vi "MNIST_Classifier(Deploy).vi"() -> ()   [LabVIEW 2024]
doc: "Overview: This example demonstrates the usage of Deep Learning Toolkit for loading the model pre-trained for handwritten digit recognition and running for inference.\nRequirements: Deep Learning Toolkit for LabVIEW."
uses:
  <vilib>/Ngene/Deep Learning Toolkit/Toolkit/NN_Network/Controls/NN_Device.ctl
  <vilib>/Ngene/Deep Learning Toolkit/Toolkit/NN_Network/Controls/NN_Save_Before_Destroy_Options.ctl
  <extravilib>/ChannelInstances/Tag-bool/Write With Abort.vi
  <extravilib>/ChannelInstances/Tag-bool/Read With Abort.vi
  <extravilib>/ChannelInstances/Tag-bool/Instantiate.vi
  <extravilib>/ChannelInstances/Tag-bool/EndpointRead.vi
  <vilib>/Ngene/Deep Learning Toolkit/Toolkit/NN_Network/API/NN_Set_Input/3D/NN_Set_Input(3D_SGL_idx).vi
  <extravilib>/ChannelInstances/Tag-bool/Endpoint.vi
  <vilib>/Ngene/Deep Learning Toolkit/Toolkit/Deep_Learning_Toolkit_by_Ngene.lvlib
  <extravilib>/ChannelInstances/Tag-bool.lvlib
panel:
  in  "Pen Width":dbl
  out "Labels":string[](array[string])=["0", "1", "2", "3", "4", "5", "6", "7", "8", "9"]
  in  "Network Configuration File Path":path
  in  "Weight File Path":path
  out "Pen Attributes":T1={"Width"=24, "Style"=enum."Solid"}
  out "Draw Digit (280x280 px)":picture
  in  "Pen Color":u32(colorbox)=197379
  in  "Clear":bool
  out "Test Speed (img/s)":dbl=2316.9601485204007 format="%#_3p"
  out "test time(s/img)":dbl=0.00043159999995623366 format="%#_3p"
  out "Predictions":sgl[](array[slide])=[0.00022317072, 0.0016224136, 0.00590554, 0.9895844, 0.0010204009, 0.00023260966, 0.00083900435, 0.00020435848, 0.00020539068, 0.00016265694] scale=0.0..1.0
  in  "Pen Width":dbl=24.0
  in  "Stop Test":bool
  out "image (28x28px)":sgl[][](graph)=[[-1.0, -1.0, -1.0, -1.0, -1.0, -1.0, -1.0, -1.0, -1.0, -1.0, -1.0, -1.0, -1.0, -1.0, -1.0, -1.0, -1.0, -1.0, -1.0, -1.0, -1.0, -1.0, -1.0, -1.0, -1.0, -1.0, -1.0, -1.0], [-1.0, -1.0, -1.0, -1.0, -1.0, -1.0, -1.0, -1.0, -1.0, -1.0, -1.0, -1.0, -1.0, -1.0, -1.0, -1.0, -1.0, -1.0, -1.0, -1.0, -1.0, -1.0, -1.0, -1.0, -1.0, -1.0, -1.0, -1.0], [-1.0, -1.0, -1.0, -1.0, -1.0, -1.0, -1.0, -1.0, -0.81929135, -0.2570866, -0.33740157, -0.6988189, -1.0, -1.0, -1.0, -1.0, -1.0, -1.0, -1.0, -1.0, -1.0, -1.0, -1.0, -1.0, -1.0, -1.0, -1.0, -1.0], [-1.0, -1.0, -1.0, -1.0, -1.0, -1.0, -1.0, -0.19685039, 0.9476378, 1.007874, 1.007874, 0.9877953, 0.024015749, -1.0, -1.0, -1.0, -1.0, -1.0, -1.0, -1.0, -1.0, -1.0, -1.0, -1.0, -1.0, -1.0, -1.0, -1.0], [-1.0, -1.0, -1.0, -1.0, -1.0, -1.0, -1.0, 0.32519686, 1.007874, 1.007874, 1.007874, 1.007874, 1.007874, -0.21692914, -1.0, -1.0, -1.0, -1.0, -1.0, -1.0, -1.0, -1.0, -1.0, -1.0, -1.0, -1.0, -1.0, -1.0], [-1.0, -1.0, -1.0, -1.0, -1.0, -1.0, -1.0, -0.81929135, -0.19685039, -0.67874014, -0.71889764, 0.72677165, 1.007874, 0.78700787, -0.9799213, -1.0, -1.0, -1.0, -1.0, -1.0, -1.0, -1.0, -1.0, -1.0, -1.0, -1.0, -1.0, -1.0], [-1.0, -1.0, -1.0, -1.0, -1.0, -1.0, -1.0, -1.0, -1.0, -1.0, -1.0, -0.2972441, 1.007874, 1.007874, -0.6586614, -1.0, -1.0, -1.0, -1.0, -1.0, -1.0, -1.0, -1.0, -1.0, -1.0, -1.0, -1.0, -1.0], [-1.0, -1.0, -1.0, -1.0, -1.0, -1.0, -1.0, -1.0, -1.0, -1.0, -1.0, -0.5984252, 1.007874, 1.007874, -0.45787403, -1.0, -1.0, -1.0, -1.0, -1.0, -1.0, -1.0, -1.0, -1.0, -1.0, -1.0, -1.0, -1.0], [-1.0, -1.0, -1.0, -1.0, -1.0, -1.0, -1.0, -1.0, -1.0, -1.0, -1.0, -0.5984252, 1.007874, 1.007874, -0.5582677, -1.0, -1.0, -1.0, -1.0, -1.0, -1.0, -1.0, -1.0, -1.0, -1.0, -1.0, -1.0, -1.0], [-1.0, -1.0, -1.0, -1.0, -1.0, -1.0, -1.0, -1.0, -1.0, -1.0, -1.0, -0.19685039, 1.007874, 1.007874, -0.6185039, -1.0, -1.0, -1.0, -1.0, -1.0, -1.0, -1.0, -1.0, -1.0, -1.0, -1.0, -1.0, -1.0], [-1.0, -1.0, -1.0, -1.0, -1.0, -1.0, -1.0, -1.0, -1.0, -1.0, -0.19685039, 0.9476378, 1.007874, 0.62637794, -0.9799213, -1.0, -1.0, -1.0, -1.0, -1.0, -1.0, -1.0, -1.0, -1.0, -1.0, -1.0, -1.0, -1.0], [-1.0, -1.0, -1.0, -1.0, -1.0, -1.0, -1.0, -0.8996063, 0.3051181, 0.72677165, 1.007874, 1.007874, 1.007874, -0.23700787, -1.0, -1.0, -1.0, -1.0, -1.0, -1.0, -1.0, -1.0, -1.0, -1.0, -1.0, -1.0, -1.0, -1.0], [-1.0, -1.0, -1.0, -1.0, -1.0, -1.0, -1.0, -0.41771653, 1.007874, 1.007874, 1.007874, 1.007874, 1.007874, 0.9677165, 0.10433071, -1.0, -1.0, -1.0, -1.0, -1.0, -1.0, -1.0, -1.0, -1.0, -1.0, -1.0, -1.0, -1.0], [-1.0, -1.0, -1.0, -1.0, -1.0, -1.0, -1.0, -0.9397638, 0.06417323, 0.20472442, 0.26496062, 0.58622044, 0.9677165, 1.007874, 1.007874, -0.056299213, -1.0, -1.0, -1.0, -1.0, -1.0, -1.0, -1.0, -1.0, -1.0, -1.0, -1.0, -1.0], [-1.0, -1.0, -1.0, -1.0, -1.0, -1.0, -1.0, -1.0, -1.0, -1.0, -1.0, -1.0, -0.75905514, 0.66653544, 1.007874, 1.007874, -0.6385827, -1.0, -1.0, -1.0, -1.0, -1.0, -1.0, -1.0, -1.0, -1.0, -1.0, -1.0], [-1.0, -1.0, -1.0, -1.0, -1.0, -1.0, -1.0, -1.0, -1.0, -1.0, -1.0, -1.0, -1.0, -0.6185039, 1.007874, 1.007874, -0.21692914, -1.0, -1.0, -1.0, -1.0, -1.0, -1.0, -1.0, -1.0, -1.0, -1.0, -1.0], [-1.0, -1.0, -1.0, -1.0, -1.0, -1.0, -1.0, -1.0, -1.0, -1.0, -1.0, -1.0, -1.0, -0.7992126, 1.007874, 1.007874, -0.39763778, -1.0, -1.0, -1.0, -1.0, -1.0, -1.0, -1.0, -1.0, -1.0, -1.0, -1.0], [-1.0, -1.0, -1.0, -1.0, -1.0, -1.0, -1.0, -1.0, -1.0, -1.0, -1.0, -1.0, -1.0, -0.036220472, 1.007874, 1.007874, -0.4980315, -1.0, -1.0, -1.0, -1.0, -1.0, -1.0, -1.0, -1.0, -1.0, -1.0, -1.0], [-1.0, -1.0, -1.0, -0.71889764, 0.36535433, -0.33740157, -1.0, -1.0, -1.0, -1.0, -1.0, -0.8996063, 0.16456693, 0.9877953, 1.007874, 0.70669293, -0.91968507, -1.0, -1.0, -1.0, -1.0, -1.0, -1.0, -1.0, -1.0, -1.0, -1.0, -1.0], [-1.0, -1.0, -1.0, 0.08425197, 1.007874, 0.9074803, -0.35748032, -0.7992126, -0.77913386, -0.45787403, 0.12440945, 0.86732286, 1.007874, 1.007874, 0.8874016, -0.6988189, -1.0, -1.0, -1.0, -1.0, -1.0, -1.0, -1.0, -1.0, -1.0, -1.0, -1.0, -1.0], [-1.0, -1.0, -1.0, -0.47795275, 0.9877953, 1.007874, 1.007874, 1.007874, 1.007874, 1.007874, 1.007874, 1.007874, 0.9877953, 0.18464567, -0.77913386, -1.0, -1.0, -1.0, -1.0, -1.0, -1.0, -1.0, -1.0, -1.0, -1.0, -1.0, -1.0, -1.0], [-1.0, -1.0, -1.0, -1.0, -0.45787403, 0.82716537, 1.007874, 1.007874, 1.007874, 1.007874, 0.9677165, 0.24488188, -0.4980315, -1.0, -1.0, -1.0, -1.0, -1.0, -1.0, -1.0, -1.0, -1.0, -1.0, -1.0, -1.0, -1.0, -1.0, -1.0], [-1.0, -1.0, -1.0, -1.0, -1.0, -0.8393701, -0.43779528, -0.39763778, -0.41771653, -0.71889764, -1.0, -1.0, -1.0, -1.0, -1.0, -1.0, -1.0, -1.0, -1.0, -1.0, -1.0, -1.0, -1.0, -1.0, -1.0, -1.0, -1.0, -1.0], [-1.0, -1.0, -1.0, -1.0, -1.0, -1.0, -1.0, -1.0, -1.0, -1.0, -1.0, -1.0, -1.0, -1.0, -1.0, -1.0, -1.0, -1.0, -1.0, -1.0, -1.0, -1.0, -1.0, -1.0, -1.0, -1.0, -1.0, -1.0], [-1.0, -1.0, -1.0, -1.0, -1.0, -1.0, -1.0, -1.0, -1.0, -1.0, -1.0, -1.0, -1.0, -1.0, -1.0, -1.0, -1.0, -1.0, -1.0, -1.0, -1.0, -1.0, -1.0, -1.0, -1.0, -1.0, -1.0, -1.0], [-1.0, -1.0, -1.0, -1.0, -1.0, -1.0, -1.0, -1.0, -1.0, -1.0, -1.0, -1.0, -1.0, -1.0, -1.0, -1.0, -1.0, -1.0, -1.0, -1.0, -1.0, -1.0, -1.0, -1.0, -1.0, -1.0, -1.0, -1.0], [-1.0, -1.0, -1.0, -1.0, -1.0, -1.0, -1.0, -1.0, -1.0, -1.0, -1.0, -1.0, -1.0, -1.0, -1.0, -1.0, -1.0, -1.0, -1.0, -1.0, -1.0, -1.0, -1.0, -1.0, -1.0, -1.0, -1.0, -1.0], [-1.0, -1.0, -1.0, -1.0, -1.0, -1.0, -1.0, -1.0, -1.0, -1.0, -1.0, -1.0, -1.0, -1.0, -1.0, -1.0, -1.0, -1.0, -1.0, -1.0, -1.0, -1.0, -1.0, -1.0, -1.0, -1.0, -1.0, -1.0]]
  # "Overview: This example demonstrates the usage of Deep Learning Toolkit for loading the model pre-trained for handwritten digit recognition and running for inference.\nRequirements: Deep Learning Toolkit for LabVIEW.\nInstructions:\nThis example requires the training results (network topology file and trained weights file) generated by MNIST_Classifier_MLP(Train).vi or MNIST_Classifier_CNN(Train).vi\n1. Provide \"Network Configuration File Path\" and \"Weight File Path\" generated from one of the examples above.\n2. Run the VI.\n3. Draw a digit on the \"Draw Digit\"  interface and observe the predictions results.\n\nMore Examples:  https://github.com/ngenehub/deepltk_examples"
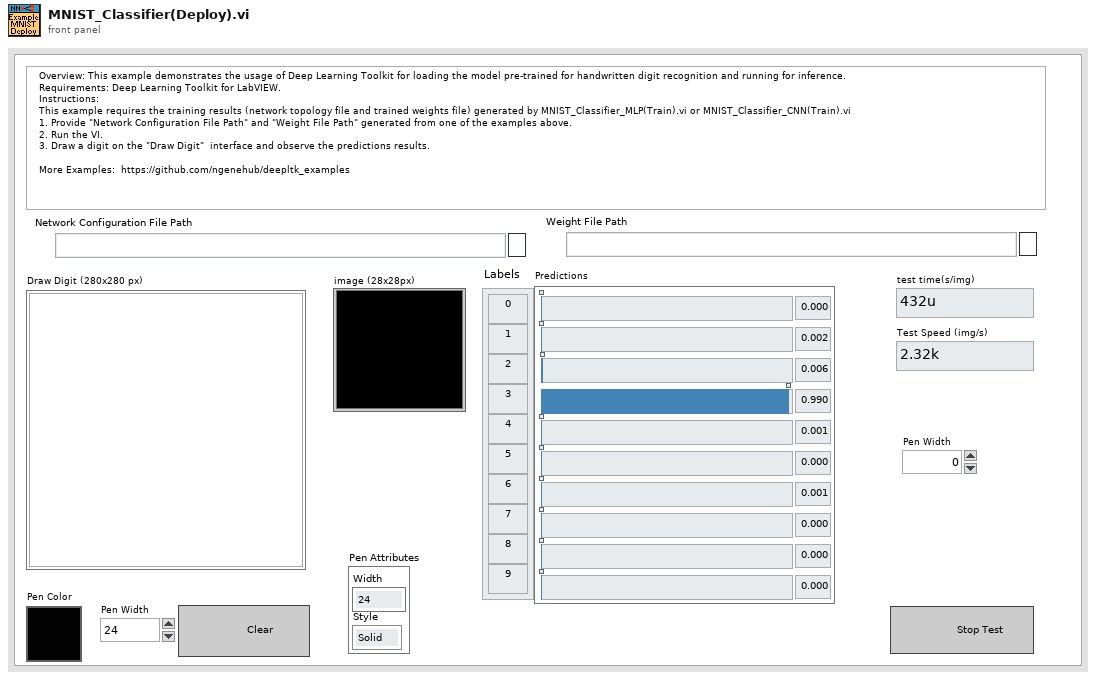
[diagram p1: front panel]
types:
  T1 = cluster{"Width":u16, "Style":enum32{"Solid", "Dash", "Dot", "DashDot", "DashDotDot"}}
  T2 = typedef "Deep_Learning_Toolkit_by_Ngene.lvlib/NN_Device.ctl" = enum16{"CPU", "GPU"}
  T3 = typedef "Deep_Learning_Toolkit_by_Ngene.lvlib/NN_Save_Before_Destroy_Options.ctl" = cluster{"CFG?":bool, "Weights?":bool, "Render?":bool}
  T4 = typedef "Deep_Learning_Toolkit_by_Ngene.lvlib/NN_Config_Params.ctl" = cluster{"Name":string, "mBatch":i32, "NN_Train_Params":T5, "LR_Decay_Policy":T8, "Labels":string[], "Loss":T10}
  T5 = typedef "Deep_Learning_Toolkit_by_Ngene.lvlib/NN_Train_Params.ctl" = cluster{"Optimizer":T6, "Beta_1":sgl, "Beta_2":sgl, "Weight Decay(L1)":sgl, "Weight Decay(L2)":sgl, "Data_Sampling":T7}
  T6 = typedef "Deep_Learning_Toolkit_by_Ngene.lvlib/NN_Train_Optimizer.ctl" = enum16{"SGD", "Adam", "Adagrad", "Adadelta", "RMSProp", "Nesterov"}
  T7 = typedef "Deep_Learning_Toolkit_by_Ngene.lvlib/NN_Train_Data_Sampling.ctl" = enum16{"Random", "Sequential"}
  T8 = typedef "Deep_Learning_Toolkit_by_Ngene.lvlib/NN_LR_Policy_Cfg.ctl" = cluster{"Policy_Type":T9, "LR0":dbl, "k":sgl, "WarmUp_Policy":enum16{"Step", "Ramp"}, "WarmUp_Iter":i32, "WarmUp_Ratio":sgl}
  T9 = typedef "Deep_Learning_Toolkit_by_Ngene.lvlib/NN_LR_Policy_Type.ctl" = enum16{"Manual", "Step", "Exp", "1/t"}
  T10 = typedef "Deep_Learning_Toolkit_by_Ngene.lvlib/NN_Loss_Config_Params.ctl" = cluster{"Loss_Type":T11, "Loss_Conf_Params":variant}
  T11 = typedef "Deep_Learning_Toolkit_by_Ngene.lvlib/NN_Loss_Type.ctl" = enum16{"None", "MSE", "CrossEntropy", "YOLO_v2", "YOLO_v4"}
  T12 = typedef "Deep_Learning_Toolkit_by_Ngene.lvlib/NN_Layer_Config_Params.ctl" = cluster{"Layer_Type":T13, "Layer_Conf_Params":variant, "Input Layers":string[]}
  T13 = typedef "Deep_Learning_Toolkit_by_Ngene.lvlib/NN_Layer_Type.ctl" = enum16{"Input1D", "Input3D", "Conv1D", "Conv2D", "Conv2D_Adv", "MaxPool", "AvgPool", "UpSample", "DropOut3D", "ShortCut", "Concat", "SoftMax3D", "FC", "DropOut", "Softmax", "Flatten", "YOLO_v2", "YOLO_v4", "Activation", "BatchNormalization", "Unsupported"}
  T14 = typedef "Deep_Learning_Toolkit_by_Ngene.lvlib/NN.ctl" = cluster{"Name":string, "No of Layers":i32, "mBatch":i32, "Layers":T15[], "Dimty":T16, "Dims_In":T17, "Dims_Out":T17, "Working_Dir":path, "Train?":bool, "Train_Params":T5, "LR_Update_Policy":T8, "Session Data":T18, "Ground_truth":T19, "NNg_hdls":T20, "NN_Device":T2, "GPU Id":i32, "Labels":string[], "Receptive Field":T21[], "Loss_Type":T11, "Loss_Cfg_Prms":variant, "NNG_WS":T22}
  T15 = typedef "Deep_Learning_Toolkit_by_Ngene.lvlib/NN_Layer_ref.ctl" = refnum<data-value>
  T16 = typedef "Deep_Learning_Toolkit_by_Ngene.lvlib/NN_In_Out_Dim-ty.ctl" = enum8{"In1D_Out1D", "In3D_Out1D", "In3D_Out3D", "In3D_OutBBox"}
  T17 = typedef "Deep_Learning_Toolkit_by_Ngene.lvlib/NN_Dims(C,H,W).ctl" = cluster{"C":i32, "H":i32, "W":i32}
  T18 = typedef "Deep_Learning_Toolkit_by_Ngene.lvlib/NN_Train_Session_Data.ctl" = cluster{"Epochs":sgl, "Tot_Iter":i32, "LR":sgl, "LR_iter":i32}
  T19 = typedef "Deep_Learning_Toolkit_by_Ngene.lvlib/NN_Ground_truth.ctl" = cluster{"Y":variant}
  T20 = typedef "Deep_Learning_Toolkit_by_Ngene.lvlib/nng_cuda_handles.ctl" = cluster{"cudnn":u64, "cublas":u64, "stream":u64, "curand":u64}
  T21 = typedef "Deep_Learning_Toolkit_by_Ngene.lvlib/NN_Dims(V,H).ctl" = cluster{"V":i32, "H":i32}
  T22 = typedef "Deep_Learning_Toolkit_by_Ngene.lvlib/NNG_WS.ctl" = cluster{"NNG_WS_Mem":T23, "Max_WS_Size":i64}
  T23 = typedef "Deep_Learning_Toolkit_by_Ngene.lvlib/NNg_WS_Mem_DVR.ctl" = refnum<data-value>
  T24 = cluster{"left":i16, "top":i16, "right":i16, "bottom":i16}
  T25 = typedef "LVMouseTypeDef.ctl" = cluster{"Mouse Position":cluster{"X":i32, "Y":i32}, "Mouse Modifiers":cluster{"Button Down":bool, "Shift Mod":bool, "Menu Mod":bool, "Option Mod":bool}}
  T26 = typedef "imagedata.ctl" = cluster{"image type":i32, "image depth":i32, "image":u8[], "mask":u8[], "colors":u32[], "Rectangle":cluster{"left":i16, "top":i16, "right":i16, "bottom":i16}}
  T27 = typedef "Tag-bool.lvlib/))Channel.ctl" = refnum<queue>
  T28 = typedef "Deep_Learning_Toolkit_by_Ngene.lvlib/NN_Layer.ctl" = cluster{"Name":string, "Layer_Data":variant, "Layer_Type":T13, "Dims_In":T17, "Layers_In":variant, "Dims_Out":T17, "Layers_Out":variant, "Metrics":T29, "GPU_Data":variant, "mBatch":i32, "NN_Device":T2, "NNg_hdls":T20, "Train?":bool, "Dimty":T30, "RecptField":T31}
  T29 = typedef "Deep_Learning_Toolkit_by_Ngene.lvlib/NN_Layer_Metrics.ctl" = cluster{"Data":dbl, "Params":dbl, "Ops":dbl}
  T30 = typedef "Deep_Learning_Toolkit_by_Ngene.lvlib/NN_Layer_Dimty.ctl" = enum16{"1D", "3D"}
  T31 = typedef "Deep_Learning_Toolkit_by_Ngene.lvlib/NN_Layer_RF_State.ctl" = cluster{"Dims":T21, "J":T21}
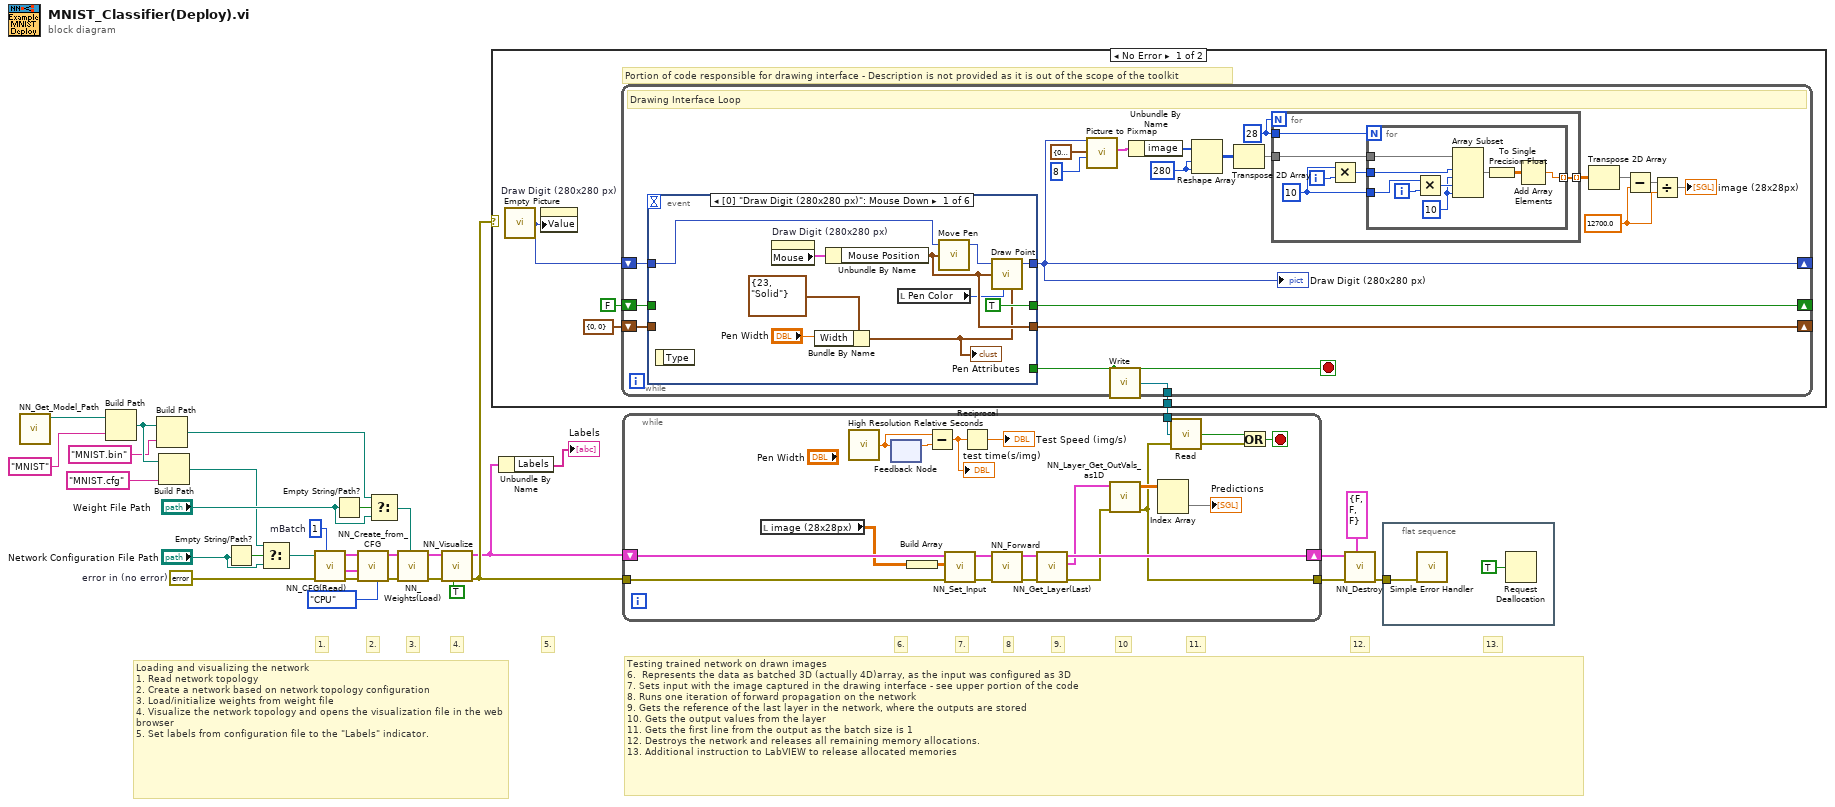
[diagram p0: block diagram]
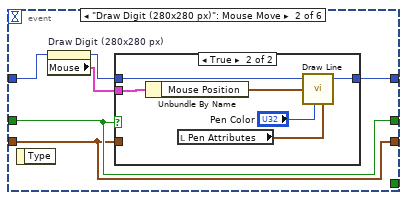
[diagram p2: hidden frame]
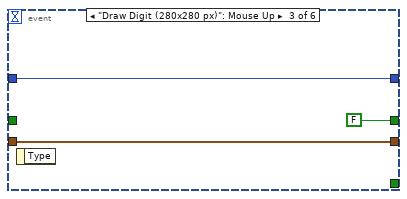
[diagram p4: hidden frame]
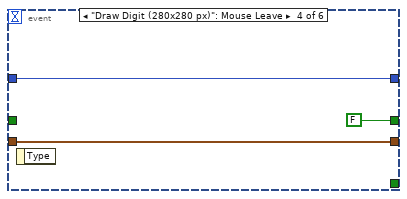
[diagram p5: hidden frame]
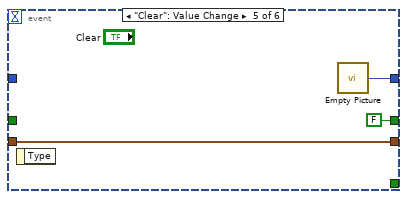
[diagram p6: hidden frame]
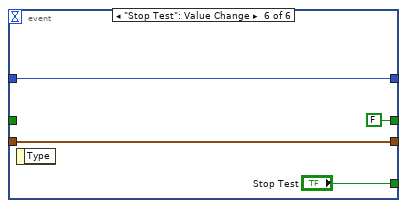
[diagram p7: hidden frame]
diagram:
  w17 = 1  # mBatch
  w24 = errorcluster {"status"=FALSE, "code"=0, "source"=""}  # error in (no error)
  # "5."
  # "Loading and visualizing the network\n1. Read network topology\n2. Create a network based on network topology configuration\n3. Load/initialize weights from weight file\n4. Visualize the network topology and opens the visualization file in the web browser\n5. Set labels from configuration file to the \"Labels\" indicator."
  # "4."
  # "3."
  # "2."
  # "1."
  # "13."
  # "12."
  # "Testing trained network on drawn images \n6.  Represents the data as batched 3D (actually 4D)array, as the input was configured as 3D\n7. Sets input with the image captured in the drawing interface - see upper portion of the code\n8. Runs one iteration of forward propagation on the network\n9. Gets the reference of the last layer in the network, where the outputs are stored\n10. Gets the output values from the layer\n11. Gets the first line from the output as the batch size is 1\n12. Destroys the network and releases all remaining memory allocations.\n13. Additional instruction to LabVIEW to release allocated memories"
  # "11."
  # "10"
  # "9."
  # "8"
  # "7."
  # "6."
  n1 = call "NN_Get_Model_Path.vi"() -> ("Model path"=w15:path)  [unwired: 11 in]
  n2 = Build Path(base path=w15, name or relative path="MNIST") -> (appended path=w13:path)
  n3 = Build Path(base path=w13, name or relative path="MNIST.bin") -> (appended path=w7:path)
  n4 = Build Path(base path=w13, name or relative path="MNIST.cfg") -> (appended path=w3:path)
  n5 = Empty String/Path?(string/path="Network Configuration File Path") -> (empty?=w6:bool)
  n6 = Select(t=w3, s=w6, f="Network Configuration File Path") -> (s? t:f=w4:path)
  n7 = call <vilib>:"NN_CFG(Read).vi"("mBatch"=w17, "error in (no error)"=w24, "CFG file path"=w4) -> ("error out"=w22:errorcluster, "Net_Cfg"=w23:T4, "Layer_Cfg"=w21:T12[])  [unwired: 6 in]
  n8 = Empty String/Path?(string/path="Weight File Path") -> (empty?=w9:bool)
  n9 = call <vilib>:"NN_Create_from_CFG.vi"("NN_Device"=NN_Device."CPU", "error in (no error)"=w22, "Net_Cfg"=w23, "Layer_Cfg"=w21) -> ("error out"=w25:errorcluster, "NN out"=w20:T14)  [unwired: 6 in]
  n10 = Select(t=w7, s=w9, f="Weight File Path") -> (s? t:f=w10:path)
  n11 = call <vilib>:"NN_Weights(Load).vi"("Weight File Path"=w10, "error in (no error)"=w25, "NN in"=w20) -> ("error out"=w26:errorcluster, "NN out"=w28:T14)  [unwired: 7 in]
  n12 = call <vilib>:"NN_Visualize.vi"("Open_in_Browser (T)"=TRUE ("Open_in_Browser"), "error in (no error)"=w26, "NN in"=w28) -> ("error out"=w19:errorcluster, "NN out"=w16:T14)  [unwired: 6 in, 1 out]
  n13 = case shown="No Error" w19 {
    tunnel: [w33 _] -> w18
    frame No Error {
      # "Portion of code responsible for drawing interface - Description is not provided as it is out of the scope of the toolkit"
      n14 = call "Empty Picture"() -> ("empty picture"=w36:picture)
      n15 = property on="Draw Digit (280x280 px)" class="Pict"("Value"=w36) -> ()  [unwired: 2 in, 2 out]
      n16 = while {
        shift-right: [w52] -> _
        shift-left: w36 -> [w57]
        shift-right: [w55] -> _
        shift-left: FALSE -> [w56]
        shift-right: [w53] -> _
        shift-left: cluster{"X":i32, "Y":i32} {"X"=0, "Y"=0} ("Mouse Position") -> [w54]
        tunnel: [w39] -> w33
        stop <- w44 stop-if-true
        w41 = sgl 12700.0 ("dimension size")
        w45 = 280 ("dimension size")
        w47 = 28
        # "Drawing Interface Loop"
        n17 = event shown="[0] \"Draw Digit (280x280 px)\": Mouse Down" {
          selector: _ -> [_ _ _ _ _ _]
          dyn-events: _ -> [_ _ _ _ _ _]
          timeout: _ -> [_ _ _ _ _ _]
          tunnel: [_ _ _ _ _ "Stop Test"] -> w44
          tunnel: [w79 w86 w97 w100 w103 w106] -> w52
          tunnel: w57 -> [w81 w85 w97 w100 _ w106]
          tunnel: w56 -> [_ w84 _ _ _ _]
          tunnel: [TRUE w84 FALSE FALSE FALSE FALSE] -> w55
          tunnel: w54 -> [_ w83 w95 w99 w102 w105]
          tunnel: [w77 w83 w95 w99 w102 w105] -> w53
          event "Draw Digit (280x280 px)": Mouse Down {
            # "Set the pen position, and draw an initial point or line."
            n18 = event-data() -> ()  [unwired: 1 in, 1 out]
            n19 = property on="Draw Digit (280x280 px)" class="Pict"() -> ("Mouse"=w82:T25)  [unwired: 2 in, 2 out]
            n20 = Bundle By Name(cluster=T1 {"Width"=23, "Style"=enum."Solid"} ("Pen Attributes"), "Width"="Pen Width") -> (w73:T1)
            "Pen Attributes" <- w73
            n21 = Unbundle By Name(w82) -> ("Mouse Position"=w77:cluster{"X":i32, "Y":i32})
            n22 = local read "Pen Color"() -> (w76:u32)
            n23 = call <vilib>:"Move Pen.vi"("new position"=w77, "picture"=w81) -> ("new picture"=w80:picture)  [unwired: 3 in]
            n24 = call <vilib>:"Draw Point.vi"("picture"=w80, "point(x,y)"=w77, "color(black)"=w76, "pen"=w73) -> ("new picture"=w79:picture)  [unwired: 5 in]
          }
          event "Draw Digit (280x280 px)": Mouse Move {
            # "Only draw if a Mouse Down event has occurred, but not a Mouse Up. Then, determine if the user is Drawing a point, a line, or selecting a subset and perform those operations in the case structure."
            n25 = event-data() -> ()  [unwired: 1 in, 1 out]
            n26 = property on="Draw Digit (280x280 px)" class="Pict"() -> ("Mouse"=w87:T25)  [unwired: 2 in, 2 out]
            n27 = case shown="True" w84 {
              tunnel: w85 -> [w88 w94]
              tunnel: w87 -> [_ w93]
              tunnel: [w88 w91] -> w86
              tunnel: w83 -> [_ _]
              frame False {
              }
              frame True {
                n28 = Unbundle By Name(w93) -> ("Mouse Position"=w92:cluster{"X":i32, "Y":i32})
                n29 = local read "Pen Attributes"() -> (w90:T1)
                n30 = call <vilib>:"Draw Line.vi"("picture"=w94, "end point"=w92, "color(black)"="Pen Color", "pen"=w90) -> ("new picture"=w91:picture)  [unwired: 5 in]
              }
            }
          }
          event "Draw Digit (280x280 px)": Mouse Up {
            # "When the user is finished drawing, we complete the operation. The only operation that we need to complete the Select Subset operation."
            n31 = event-data() -> ()  [unwired: 1 in, 1 out]
          }
          event "Draw Digit (280x280 px)": Mouse Leave {
            # "Change to the default cursor when the mouse leaves the picture."
            n32 = event-data() -> ()  [unwired: 1 in, 1 out]
          }
          event "Clear": Value Change {
            # "Erase the picture."
            n33 = event-data() -> ()  [unwired: 1 in, 1 out]
            n34 = call "Empty Picture"() -> ("empty picture"=w103:picture)
          }
          event "Stop Test": Value Change {
            # "Stop the VI."
            n35 = event-data() -> ()  [unwired: 1 in, 1 out]
          }
        }
        "Draw Digit (280x280 px)" <- w52
        n36 = call <vilib>:"Picture to Pixmap.vi"("depth"=8, "rect"=T24 {"left"=0, "top"=0, "right"=280, "bottom"=280}, "picture"=w52) -> ("image data"=w51:T26)  [unwired: 7 in, 1 out]
        n37 = call <extravilib>:"Write.vi"("element"=w44) -> ("channel"=w39:T27)  [unwired: 1 out]
        n38 = Unbundle By Name(w51) -> ("image"=w50:u8[])
        n39 = Reshape Array(w50, w45, w45) -> (w49:u8[][])
        n40 = Transpose 2D Array(2D array=w49) -> (transposed array=w48:u8[][])
        n41 = for {
          N: w47 -> [_]
          tunnel: w48 -> [w63]
          tunnel: w47 -> [w62]
          tunnel: [w58] -> w46 mode=indexing
          i -> [w61]
          w59 = 10 ("x")
          n42 = Multiply(x=w59, y=w61) -> (x*y=w60:i32)
          n43 = for {
            N: w62 -> [_]
            tunnel: w63 -> [w72]
            tunnel: w60 -> [w71]
            tunnel: w59 -> [w68]
            tunnel: [w64] -> w58 mode=indexing
            i -> [w70]
            w67 = 10 ("length")
            n44 = Multiply(x=w68, y=w70) -> (x*y=w69:i32)
            n45 = Array Subset(array=w72, index (row)=w71, length (row)=w67, index (col)=w69, length (col)=w67) -> (w66:u8[][])
            n46 = To Single Precision Float(number=w66) -> (single precision float=w65:sgl[][])
            n47 = Add Array Elements(numeric array=w65) -> (sum=w64:sgl)
          }
        }
        n48 = Transpose 2D Array(2D array=w46) -> (transposed array=w42:sgl[][])
        n49 = Subtract(x=w42, y=w41) -> (x-y=w43:sgl[][])
        n50 = Divide(x=w43, y=w41) -> (x/y=→"image (28x28px)":sgl[][])
      }
    }
    frame Error {
    }
  }
  n51 = Unbundle By Name(w16) -> ("Labels"=→"Labels":string[])
  n52 = while {
    shift-right: [w127] -> w31
    shift-left: w16 -> [w120]
    tunnel: w19 -> [w118]
    tunnel: [w111] -> w30
    tunnel: w18 -> [w110]
    stop <- w125 stop-if-true
    n53 = local read "image (28x28px)"() -> (w116:sgl[][])
    n54 = call <vilib>:"High Resolution Relative Seconds.vi"() -> ("relative seconds"=w123:dbl)
    n55 = feedback #1() -> (w124:dbl)  [unwired: 1 in]
    n56 = feedback-in #1(w123) -> ()
    n57 = Build Array(w116) -> (w108:sgl[][][])
    n58 = Subtract(x=w123, y=w124) -> (x-y=w122:dbl)
    "test time(s/img)" <- w122
    n59 = call-poly <vilib>:"NN_Set_Input.vi"("error in (no error)"=w118, "Data_In(3D_SGL)"=w108, "NN in"=w120) -> ("error out"=w117:errorcluster, "NN out"=w119:T14)  [unwired: 7 in]
    n60 = Reciprocal(x=w122) -> (1/x=→"Test Speed (img/s)":dbl)
    n61 = call <vilib>:"NN_Forward.vi"("error in (no error)"=w117, "NN in"=w119) -> ("error out"=w126:errorcluster, "NN out"=w128:T14)  [unwired: 6 in, 2 out]
    n62 = call <vilib>:"NN_Get_Layer(Last).vi"("error in (no error)"=w126, "NN in"=w128) -> ("error out"=w112:errorcluster, "Last_Layer"=w115:T28, "NN out"=w127:T14)  [unwired: 6 in, 1 out]
    n63 = call <vilib>:"NN_Layer_Get_OutVals_as1D.vi"("error in (no error)"=w112, "Layer"=w115) -> ("error out"=w111:errorcluster, "Out(as1D)"=w114:sgl[][])  [unwired: 8 in]
    n64 = Index Array(array=w114) -> (element=→"Predictions":sgl[])  [unwired: 2 in]
    n65 = call <extravilib>:"Read.vi"("channel"=w110) -> ("element"=w109:bool)  [unwired: 1 in, 1 out]
    n66 = Or(x=w109, y=w111) -> (x .or. y?=w125:bool)
  }
  n67 = call <vilib>:"NN_Destroy.vi"("Save (T, T, T)"=T3 {"CFG?"=FALSE, "Weights?"=FALSE, "Render?"=FALSE} ("Save_Config"), "error in (no error)"=w30, "NN in"=w31) -> ("error out"=w32:errorcluster)  [unwired: 7 in, 1 out]
  n68 = flat-sequence {
    tunnel: w32 -> [w130]
    frame #0 {
      n69 = call <vilib>:"Simple Error Handler.vi"("error in (no error)"=w130) -> ()  [unwired: 4 in, 5 out]
      n70 = Request Deallocation(TRUE ("flag")) -> ()
    }
  }
